vi "WriteLogEntry.vi"(0 "Path In":path, 1 "Curr Param":dbl[](array[numeric]) caption="Current Parameters", 2 "Delimiter":string, 3 "error in (no error)":errorcluster) -> (8 "error out":errorcluster)   [LabVIEW 2009]
doc: "Writes a 1D array of doubles as a line in a log entry, with default delimiter (\\t)"
uses:
  <vilib>/Utility/file.llb/Write To Spreadsheet File (DBL).vi
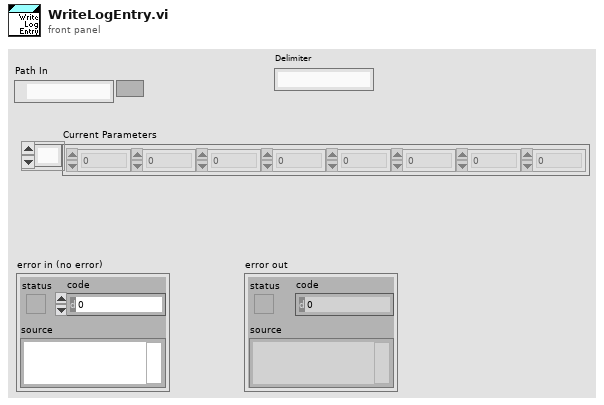
[diagram p1: front panel]
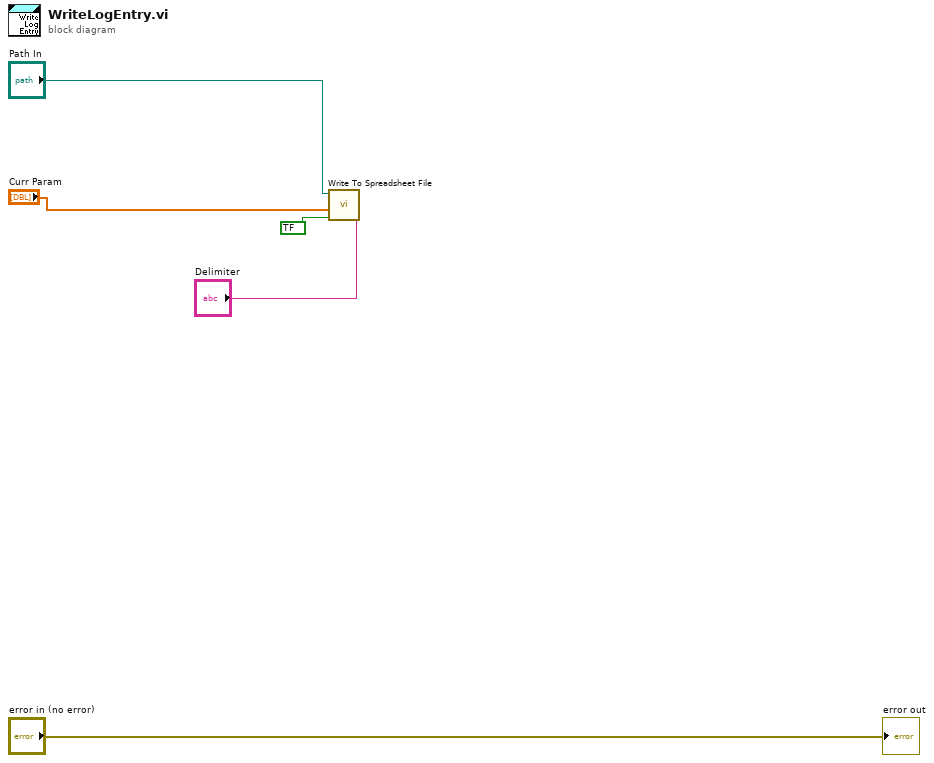
[diagram p0: block diagram]
diagram:
  n1 = call-poly <vilib>:"Write To Spreadsheet File.vi"("delimiter (\\t)"="Delimiter", "append to file? (new file:F)"=bool ?, "1D data"="Curr Param", "file path (dialog if empty)"="Path In") -> ()  [unwired: 4 in, 1 out]
  "error out" <- "error in (no error)"
